vi "VI Tree.vi"   [LabVIEW 2021, in "Environment Chamber.lvlib" / "Climatic Chamber.lvlib"]
doc: "This is the instrument driver for the <INSTRUMENT NAME>. The VI Tree displays all the user-callable VIs of the instrument driver in an organized table."
uses:
  Climatic Chamber.lvlib
  Action-Status/Timer/Status TimerList (Quick).vi
  Action-Status/Specimen/Status SpecimenTempCtrlSettings(P).vi
  Data/Monitor ConstantSet (Temp).vi
  Action-Status/Timer/Set Timer (Quick).vi
panel:
  # "(c) 2015 <Espec Corp.>.  ALL RIGHTS RESERVED."
  # "SEE DIAGRAM\nFOR VI TREE."
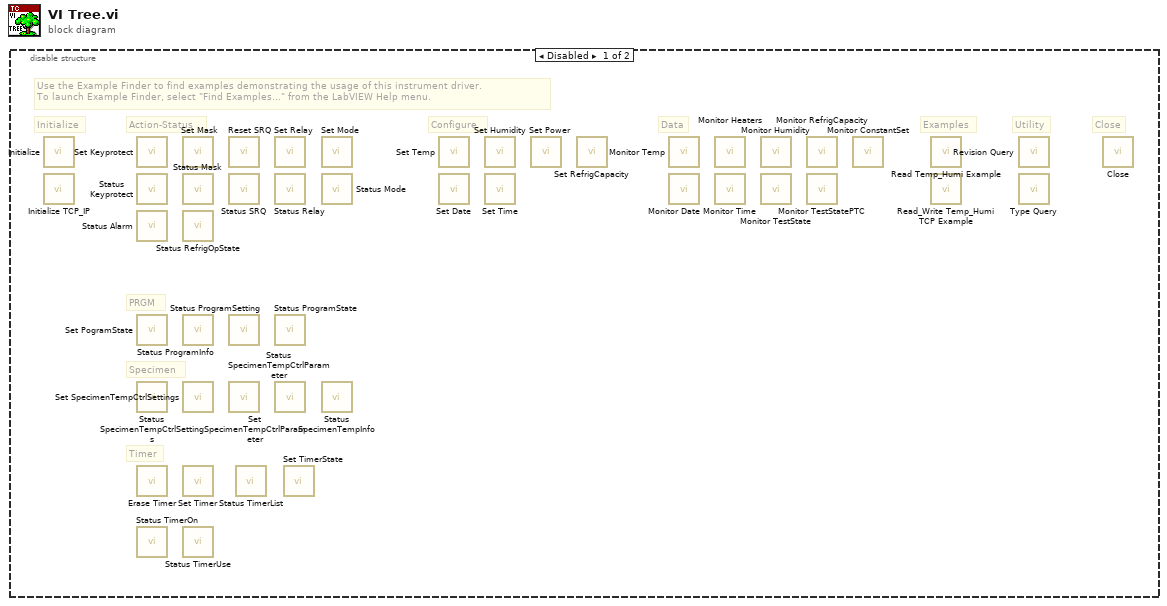
[diagram p0: block diagram]
diagram:
  n1 = disable-structure shown="Disabled" {
    frame Disabled {
      # "Close"
      # "Utility"
      # "Examples"
      # "Data"
      # "Configure"
      # "Timer"
      # "Specimen"
      # "PRGM"
      # "Action-Status"
      # "Initialize"
      # "Use the Example Finder to find examples demonstrating the usage of this instrument driver.\nTo launch Example Finder, select \"Find Examples...\" from the LabVIEW Help menu."
      n2 = call "Initialize.vi"() -> ()  [unwired: 10 in, 2 out]
      n3 = call "Initialize TCP_IP.vi"() -> ()  [unwired: 10 in, 2 out]
      n4 = call "Set Keyprotect.vi"() -> ()  [unwired: 10 in, 2 out]
      n5 = call "Status Keyprotect.vi"() -> ()  [unwired: 9 in, 3 out]
      n6 = call "Status Alarm.vi"() -> ()  [unwired: 8 in, 4 out]
      n7 = call "Set PogramState.vi"() -> ()  [unwired: 9 in, 3 out]
      n8 = call-poly "Status SpecimenTempCtrlSettings.vi"() -> ()  [unwired: 7 in, 5 out]
      n9 = call "Erase Timer.vi"() -> ()  [unwired: 10 in, 2 out]
      n10 = call "Status TimerOn.vi"() -> ()  [unwired: 8 in, 4 out]
      n11 = call "Set Mask.vi"() -> ()  [unwired: 10 in, 2 out]
      n12 = call "Status Mask.vi"() -> ()  [unwired: 8 in, 4 out]
      n13 = call "Status RefrigOpState.vi"() -> ()  [unwired: 8 in, 4 out]
      n14 = call "Status ProgramInfo.vi"() -> ()  [unwired: 6 in, 6 out]
      n15 = call "Set SpecimenTempCtrlSettings.vi"() -> ()  [unwired: 10 in, 2 out]
      n16 = call-poly "Set Timer.vi"() -> ()  [unwired: 10 in, 2 out]
      n17 = call "Status TimerUse.vi"() -> ()  [unwired: 8 in, 4 out]
      n18 = call "Reset SRQ.vi"() -> ()  [unwired: 10 in, 2 out]
      n19 = call "Status SRQ.vi"() -> ()  [unwired: 8 in, 4 out]
      n20 = call "Status ProgramSetting.vi"() -> ()  [unwired: 7 in, 5 out]
      n21 = call "Status SpecimenTempCtrlParameter.vi"() -> ()  [unwired: 9 in, 3 out]
      n22 = call-poly "Status TimerList.vi"() -> ()  [unwired: 9 in, 3 out]
      n23 = call "Set Relay.vi"() -> ()  [unwired: 10 in, 2 out]
      n24 = call "Status Relay.vi"() -> ()  [unwired: 8 in, 4 out]
      n25 = call "Status ProgramState.vi"() -> ()  [unwired: 9 in, 3 out]
      n26 = call "Set SpecimenTempCtrlParameter.vi"() -> ()  [unwired: 10 in, 2 out]
      n27 = call "Set TimerState.vi"() -> ()  [unwired: 10 in, 2 out]
      n28 = call "Set Mode.vi"() -> ()  [unwired: 10 in, 2 out]
      n29 = call "Status Mode.vi"() -> ()  [unwired: 9 in, 3 out]
      n30 = call "Status SpecimenTempInfo.vi"() -> ()  [unwired: 8 in, 4 out]
      n31 = call "Set Temp.vi"() -> ()  [unwired: 10 in, 2 out]
      n32 = call "Set Date.vi"() -> ()  [unwired: 10 in, 2 out]
      n33 = call "Set Humidity.vi"() -> ()  [unwired: 10 in, 2 out]
      n34 = call "Set Time.vi"() -> ()  [unwired: 10 in, 2 out]
      n35 = call "Set Power.vi"() -> ()  [unwired: 10 in, 2 out]
      n36 = call "Set RefrigCapacity.vi"() -> ()  [unwired: 10 in, 2 out]
      n37 = call "Monitor Temp.vi"() -> ()  [unwired: 6 in, 6 out]
      n38 = call "Monitor Date.vi"() -> ()  [unwired: 7 in, 5 out]
      n39 = call "Monitor Heaters.vi"() -> ()  [unwired: 7 in, 5 out]
      n40 = call "Monitor Time.vi"() -> ()  [unwired: 6 in, 6 out]
      n41 = call "Monitor Humidity.vi"() -> ()  [unwired: 6 in, 6 out]
      n42 = call "Monitor TestState.vi"() -> ()  [unwired: 6 in, 6 out]
      n43 = call "Monitor RefrigCapacity.vi"() -> ()  [unwired: 8 in, 4 out]
      n44 = call "Monitor TestStatePTC.vi"() -> ()  [unwired: 5 in, 7 out]
      n45 = call-poly "Monitor ConstantSet.vi"() -> ()  [unwired: 9 in, 3 out]
      n46 = call "Read Temp_Humi Example.vi"() -> ()  [unwired: 12 in]
      n47 = call "Read_Write Temp_Humi TCP Example.vi"() -> ()  [unwired: 12 in]
      n48 = call "Revision Query.vi"() -> ()  [unwired: 8 in, 4 out]
      n49 = call "Type Query.vi"() -> ()  [unwired: 9 in, 3 out]
      n50 = call "Close.vi"() -> ()  [unwired: 11 in, 1 out]
    }
    frame Enabled {
    }
  }
